vi "test.vi"() -> ()   [LabVIEW 2016]
uses:
  ti2_lightPath.ctl
  ti2_filterPos.ctl
  ti2lv.lvlib
panel:
  out "pUserOutParam":i32[](array[numeric])
  in  "Filter Position Set":T1=1 items=["1"=1, "2"=2, "3"=3, "4"=4, "5"=5, "6"=6]
  out "Filter Position":T1=1 items=["1"=1, "2"=2, "3"=3, "4"=4, "5"=5, "6"=6]
  in  "Light Path Set":T2=1 items=["Eyepieces"=1, "Right"=2, "Bottom"=3, "Left"=4]
  in  "z Position Set (um)":dbl
  out "Light Path":T2=1 items=["Eyepieces"=1, "Right"=2, "Bottom"=3, "Left"=4]
  out "z Position (um)":dbl
  in  "Stop":bool
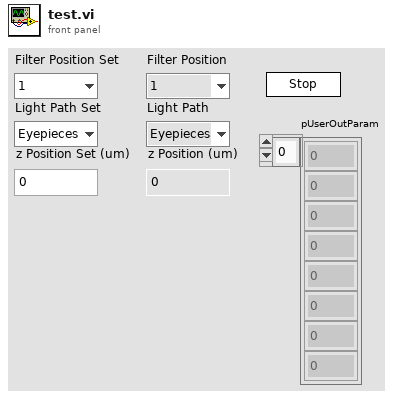
[diagram p1: front panel]
types:
  T1 = typedef "ti2lv.lvlib/ti2_filterPos.ctl" = u16
  T2 = typedef "ti2lv.lvlib/ti2_lightPath.ctl" = i32
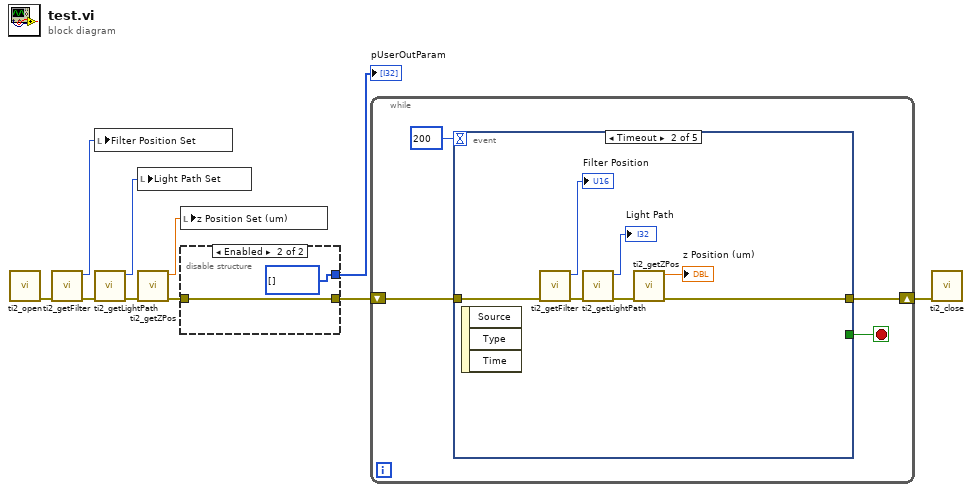
[diagram p0: block diagram]
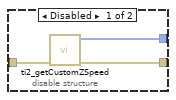
[diagram p2: hidden frame]
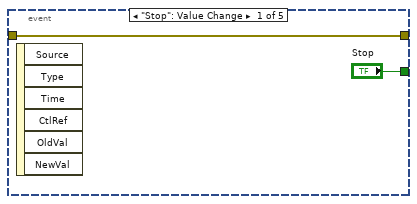
[diagram p3: hidden frame]
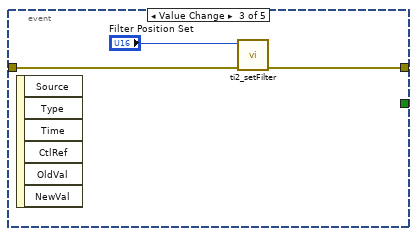
[diagram p4: hidden frame]
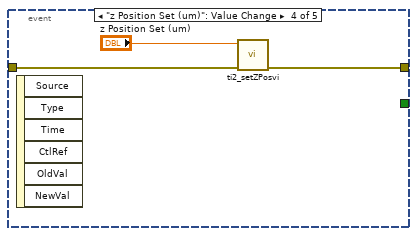
[diagram p5: hidden frame]
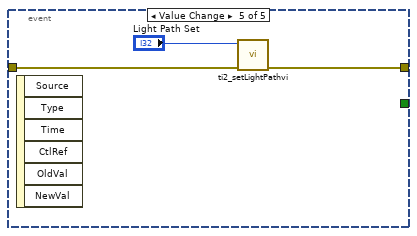
[diagram p6: hidden frame]
diagram:
  n1 = call "ti2_open.vi"() -> ("error out"=w7:errorcluster)  [unwired: 11 in]
  n2 = call "ti2_getFilter.vi"("error in (no error)"=w7) -> ("error out"=w8:errorcluster, "Filter Position"=w6:T1)  [unwired: 9 in]
  n3 = local write "Filter Position Set"(w6) -> ()
  n4 = call "ti2_getLightPath.vi"("error in (no error)"=w8) -> ("error out"=w9:errorcluster, "Light Path"=w5:T2)  [unwired: 9 in]
  n5 = local write "Light Path Set"(w5) -> ()
  n6 = call "ti2_getZPos.vi"("error in (no error)"=w9) -> ("error out"=w3:errorcluster, "z Position (um)"=w4:dbl)  [unwired: 9 in]
  n7 = local write "z Position Set (um)"(w4) -> ()
  n8 = disable-structure shown="Enabled" {
    disable-tunnel: w3 -> [w13 w15]
    disable-tunnel: [w12 w15] -> w2
    disable-tunnel: [w11 i32[] [] ("pUserOutParam")] -> w1
    frame Disabled {
      n9 = call "ti2_getCustomZSpeed.vi"("error in (no error)"=w13) -> ("error out"=w12:errorcluster, "pUserOutParam"=w11:i32[])  [unwired: 9 in]
    }
    frame Enabled {
    }
  }
  "pUserOutParam" <- w1
  n10 = while {
    shift-right: [w17] -> w10
    shift-left: w2 -> [w18]
    stop <- w19 stop-if-true
    n11 = event shown="[1] Timeout" {
      selector: _ -> [_ _ _ _ _]
      dyn-events: _ -> [_ _ _ _ _]
      timeout: 200 -> [_ _ _ _ _]
      tunnel: ["Stop" _ _ _ _] -> w19
      tunnel: w18 -> [w20 w28 w31 w34 w37]
      tunnel: [w20 w25 w30 w32 w36] -> w17
      event "Stop": Value Change {
        n12 = event-data() -> ()  [unwired: 1 in, 6 out]
      }
      event Timeout {
        n13 = event-data() -> ()  [unwired: 1 in, 3 out]
        n14 = call "ti2_getFilter.vi"("error in (no error)"=w28) -> ("error out"=w27:errorcluster, "Filter Position"=→"Filter Position":T1)  [unwired: 9 in]
        n15 = call "ti2_getLightPath.vi"("error in (no error)"=w27) -> ("error out"=w26:errorcluster, "Light Path"=→"Light Path":T2)  [unwired: 9 in]
        n16 = call "ti2_getZPos.vi"("error in (no error)"=w26) -> ("error out"=w25:errorcluster, "z Position (um)"=→"z Position (um)":dbl)  [unwired: 9 in]
      }
      event Value Change {
        n17 = event-data() -> ()  [unwired: 1 in, 6 out]
        n18 = call "ti2_setFilter.vi"("error in (no error)"=w31, "Filter Position"="Filter Position Set") -> ("error out"=w30:errorcluster)  [unwired: 9 in]
      }
      event "z Position Set (um)": Value Change {
        n19 = event-data() -> ()  [unwired: 1 in, 6 out]
        n20 = call "ti2_setZPosvi.vi"("error in (no error)"=w34, "z Position (um)"="z Position Set (um)") -> ("error out"=w32:errorcluster)  [unwired: 9 in]
      }
      event Value Change {
        n21 = event-data() -> ()  [unwired: 1 in, 6 out]
        n22 = call "ti2_setLightPathvi.vi"("error in (no error)"=w37, "Light Path"="Light Path Set") -> ("error out"=w36:errorcluster)  [unwired: 9 in]
      }
    }
  }
  n23 = call "ti2_close.vi"("error in (no error)"=w10) -> ()  [unwired: 10 in, 1 out]
